vi "AutoDrawBackground.vi"(1 "File Path":path) -> (0 "File Path Out":path)   [LabVIEW 2017]
uses:
  <vilib>/vision/NI_Vision_Development_Module.lvlib
panel:
  in  "ScaleFactor":i32=1
  out "Image":T1(plugin-control)
  in  "Scale":u32(colorbox)=9868950
  in  "Platform":u32(colorbox)=13816530
  in  "Switch":u32(colorbox)=9868950
  in  "Auto Line":u32(colorbox)=13816530
  in  "Pyramid":u32(colorbox)=12369084
  in  "Exchange":u32(colorbox)=12369084
  in  "Perimeter":u32(colorbox)
  in  "Scale (in)":cluster{"X":dbl, "Y":dbl}[](array[cluster])=[{"X"=299.65, "Y"=71.57}, {"X"=348.35, "Y"=71.57}, {"X"=348.35, "Y"=107.57}, {"X"=330.0, "Y"=107.57}, {"X"=330.0, "Y"=216.43}, {"X"=348.35, "Y"=216.43}, {"X"=348.35, "Y"=252.43}, {"X"=299.65, "Y"=252.43}, {"X"=299.65, "Y"=216.43}, {"X"=318.0, "Y"=216.43}, {"X"=318.0, "Y"=107.57}, {"X"=299.65, "Y"=107.57}, {"X"=299.65, "Y"=71.57}]
  in  "Platform (in)":cluster{"X":dbl, "Y":dbl}[](array[cluster])=[{"X"=261.47, "Y"=95.25}, {"X"=386.53, "Y"=95.25}, {"X"=386.53, "Y"=228.75}, {"X"=261.47, "Y"=228.75}, {"X"=261.47, "Y"=95.25}]
  in  "Switch (in)":cluster{"X":dbl, "Y":dbl}[](array[cluster])=[{"X"=140.0, "Y"=85.25}, {"X"=196.0, "Y"=85.25}, {"X"=196.0, "Y"=238.75}, {"X"=140.0, "Y"=238.75}, {"X"=140.0, "Y"=85.25}]
  in  "Auto Line (in)":cluster{"X":dbl, "Y":dbl}[](array[cluster])=[{"X"=120.0, "Y"=0.0}, {"X"=120.0, "Y"=324.0}]
  in  "Pyramid (in)":cluster{"X":dbl, "Y":dbl}[](array[cluster])=[{"X"=140.0, "Y"=139.5}, {"X"=98.0, "Y"=139.5}, {"X"=98.0, "Y"=184.5}, {"X"=140.0, "Y"=184.5}]
  in  "Exchange (in)":cluster{"X":dbl, "Y":dbl}[](array[cluster])=[{"X"=0.0, "Y"=174.0}, {"X"=36.0, "Y"=174.0}, {"X"=36.0, "Y"=222.0}, {"X"=0.0, "Y"=222.0}]
  in  "Field Perimeter (in)":cluster{"X":dbl, "Y":dbl}[](array[cluster])=[{"X"=648.0, "Y"=29.69}, {"X"=613.0, "Y"=0.0}, {"X"=35.0, "Y"=0.0}, {"X"=0.0, "Y"=29.69}, {"X"=0.0, "Y"=294.31}, {"X"=35.0, "Y"=324.0}, {"X"=613.0, "Y"=324.0}, {"X"=648.0, "Y"=294.31}]
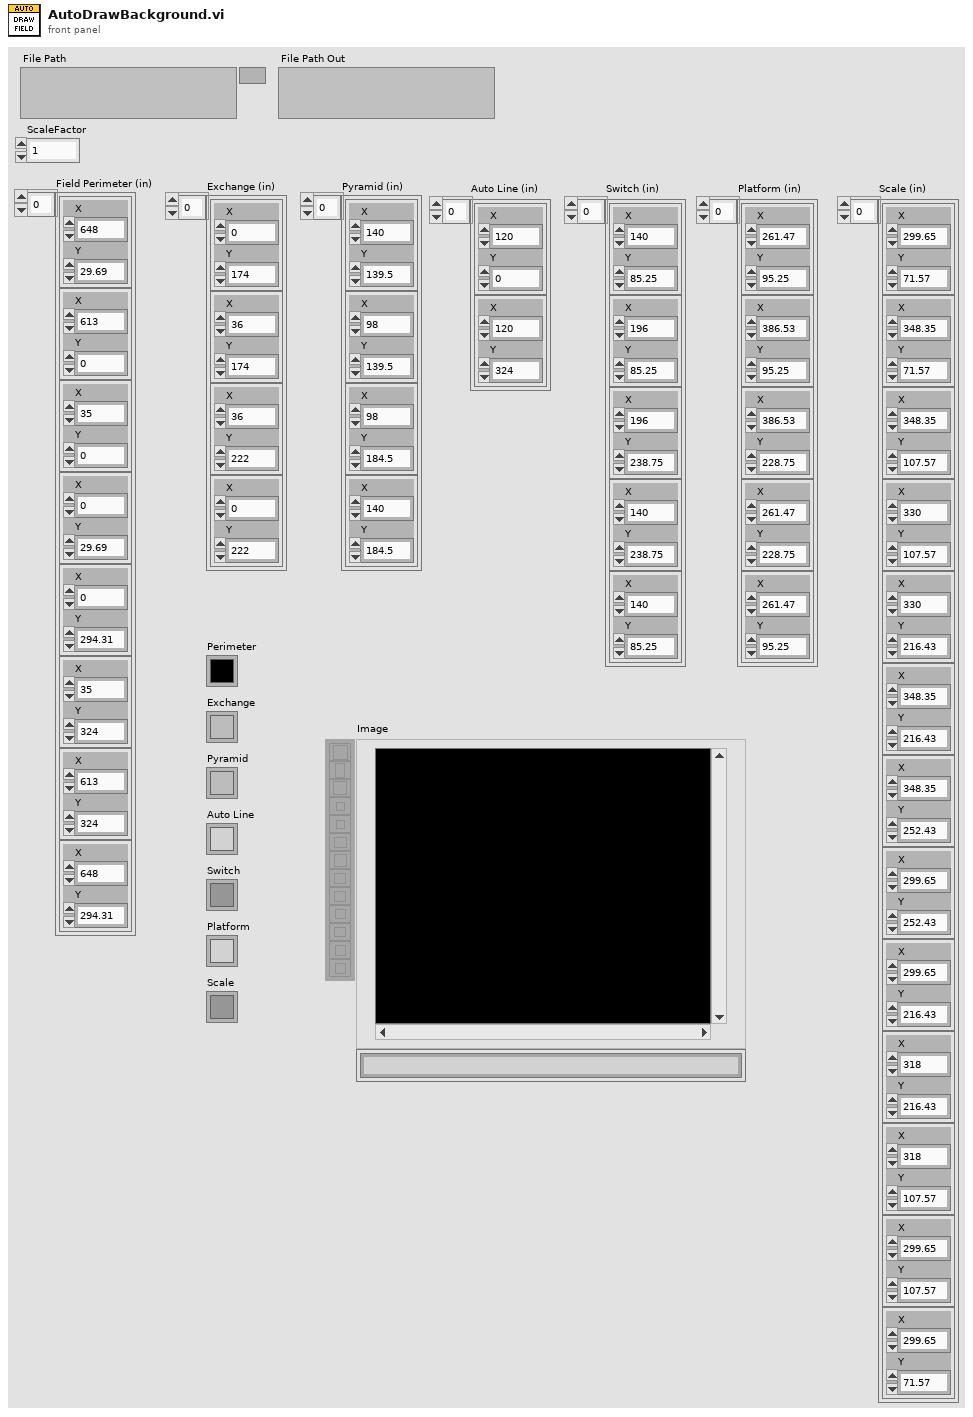
[diagram p1: front panel]
types:
  T1 = typedef "IMAQ Image.ctl" = refnum<image>
  T2 = typedef "Image Type" = u32
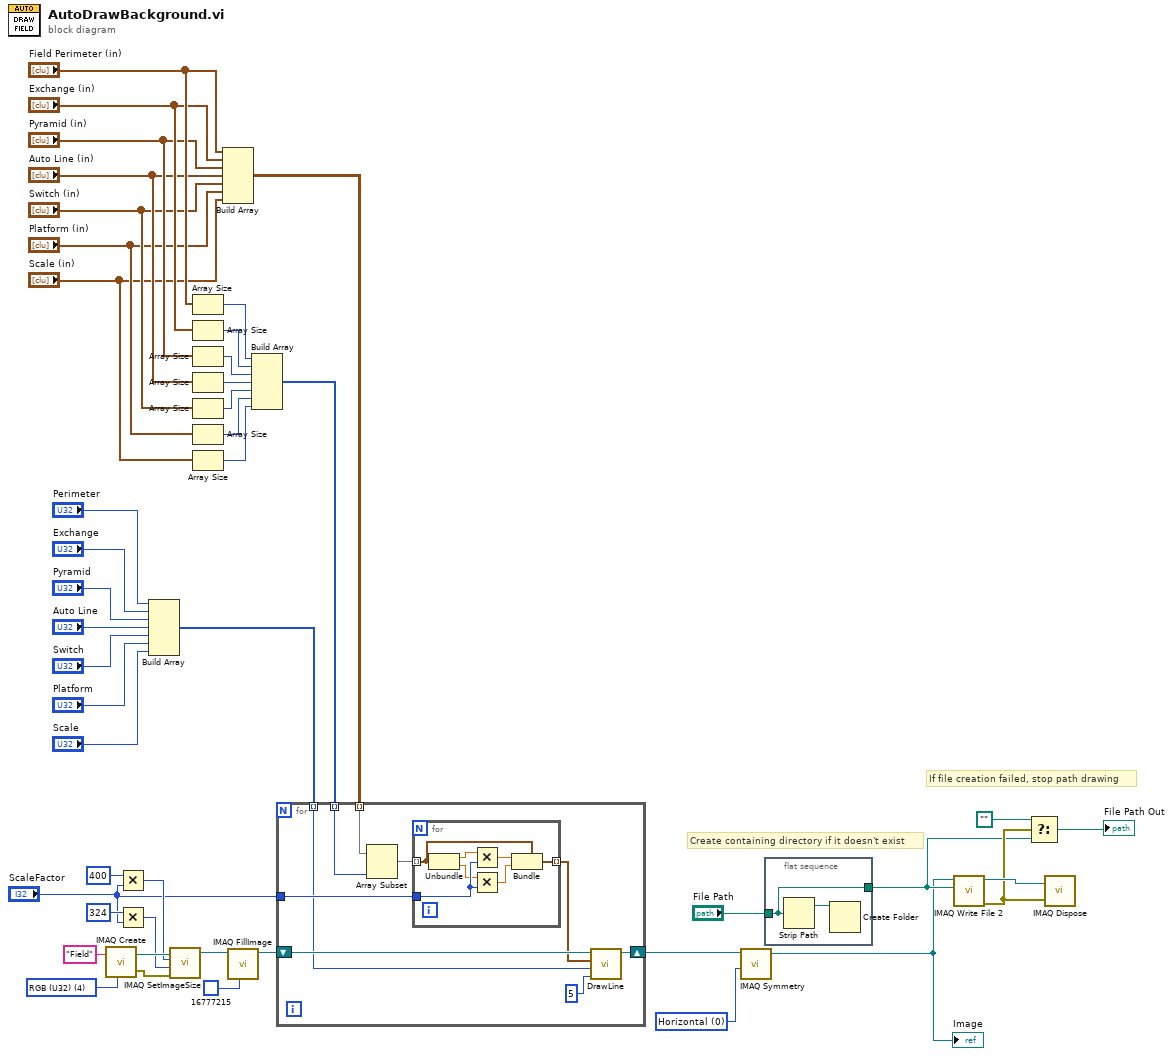
[diagram p0: block diagram]
diagram:
  w11 = u32 0 items=["Horizontal", "Vertical", "Central", "1st Diagonal", "2nd Diagonal"] ("Type of Symmetry")
  w43 = T2 4 items=["Grayscale (U8)", "Grayscale (I16)", "Grayscale (SGL)", "Complex (CSG)", "RGB (U32)", "HSL (U32)", "RGB (U64)", "Grayscale (U16)"] ("Image Type")
  # "Create containing directory if it doesn't exist"
  # "If file creation failed, stop path drawing"
  n1 = call "IMAQ Create"("Image Name"="Field", "Image Type"=w43) -> ("New Image"=w44:T1, "error out"=w45:errorcluster)  [unwired: 3 in]
  n2 = Multiply(x=400 ("X Resolution"), y="ScaleFactor") -> (x*y=w14:i32)
  n3 = Multiply(x=324 ("Y Resolution"), y="ScaleFactor") -> (x*y=w13:i32)
  n4 = Build Array("Perimeter", "Exchange", "Pyramid", "Auto Line", "Switch", "Platform", "Scale") -> (w33:u32[])
  n5 = call "IMAQ SetImageSize"("error in (no error)"=w45, "Y Resolution"=w13, "X Resolution"=w14, "Image"=w44) -> ("Image Out"=w2:T1)  [unwired: 1 in, 1 out]
  n6 = Array Size(array="Field Perimeter (in)") -> (size(s)=w25:i32)
  n7 = Array Size(array="Exchange (in)") -> (size(s)=w23:i32)
  n8 = Array Size(array="Pyramid (in)") -> (size(s)=w21:i32)
  n9 = Array Size(array="Auto Line (in)") -> (size(s)=w19:i32)
  n10 = Array Size(array="Switch (in)") -> (size(s)=w20:i32)
  n11 = Array Size(array="Platform (in)") -> (size(s)=w22:i32)
  n12 = Array Size(array="Scale (in)") -> (size(s)=w24:i32)
  n13 = Build Array("Field Perimeter (in)", "Exchange (in)", "Pyramid (in)", "Auto Line (in)", "Switch (in)", "Platform (in)", "Scale (in)") -> (w34:cluster{"X":dbl, "Y":dbl}[][])
  n14 = call "IMAQ FillImage"("Color Pixel Value"=u32 16777215, "Image"=w2) -> ("Image Out"=w3:T1)  [unwired: 8 in, 1 out]
  n15 = Build Array(w25, w23, w21, w19, w20, w22, w24) -> (w18:i32[])
  n16 = for {
    shift-right: [w49] -> w5
    shift-left: w3 -> [w50]
    tunnel: w34 -> [w54] mode=indexing
    tunnel: w33 -> [w47] mode=indexing
    tunnel: w18 -> [w53] mode=indexing
    tunnel: "ScaleFactor" -> [w51]
    n17 = Array Subset(array=w54, length=w53) -> (w52:cluster{"X":dbl, "Y":dbl}[])  [unwired: 1 in]
    n18 = for {
      tunnel: w52 -> [w56] mode=indexing
      tunnel: w51 -> [w61]
      tunnel: [w55] -> w48 mode=indexing
      n19 = Unbundle(w56) -> ("X"=w60:dbl, "Y"=w59:dbl)
      n20 = Multiply(x=w60, y=w61) -> (x*y=w58:dbl)
      n21 = Multiply(x=w59, y=w61) -> (x*y=w57:dbl)
      n22 = Bundle(cluster=w56, "X"=w58, "Y"=w57) -> (w55:cluster{"X":dbl, "Y":dbl})
    }
    n23 = call "DrawLine.vi"("Line Width (px)"=u8 5 ("Width"), "Color"=w47, "Line Endpoints"=w48, "Image"=w50) -> ("Image Out"=w49:T1)  [unwired: 7 in]
  }
  n24 = call "IMAQ Symmetry"("Type of Symmetry"=w11, "Image Src"=w5) -> ("Image Dst Out"=w4:T1)  [unwired: 3 in, 1 out]
  "Image" <- w4
  n25 = flat-sequence {
    tunnel: "File Path" -> [w62]
    tunnel: [w62] -> w6
    frame #0 {
      n26 = Strip Path(path=w62) -> (stripped path=w63:path)  [unwired: 1 out]
      n27 = Create Folder(path (use dialog)=w63) -> ()  [unwired: 2 in, 3 out]
    }
  }
  n28 = call-poly "IMAQ Write File 2"("File Path"=w6, "Image"=w4) -> ("error out"=w10:errorcluster, "Image Out (duplicate)"=w17:T1)  [unwired: 8 in]
  n29 = Select(t=path "", s=w10, f=w6) -> (s? t:f=→"File Path Out":path)
  n30 = call "IMAQ Dispose"("Image"=w17, "error in (no error)"=w10) -> ()  [unwired: 4 in, 1 out]
